vi "Lock Graph Legend in The TopRight.vi"(6 "offset":cluster{"x":i32, "y":i32}, 8 "error in (no error)":errorcluster, 11 "TabControl in":refnum<vi>) -> (0 "error out":errorcluster)   [LabVIEW 2017]
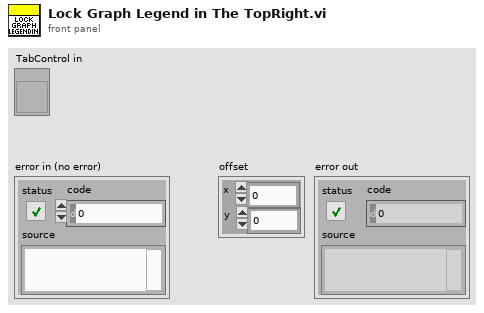
[diagram p1: front panel]
types:
  T1 = typedef "LVBoundsTypeDef.ctl" = cluster{"Width":u32, "Height":u32}
  T2 = typedef "LVPositionTypeDef.ctl" = cluster{"Left":i32, "Top":i32}
  T3 = cluster{"left":i16, "top":i16, "right":i16, "bottom":i16}
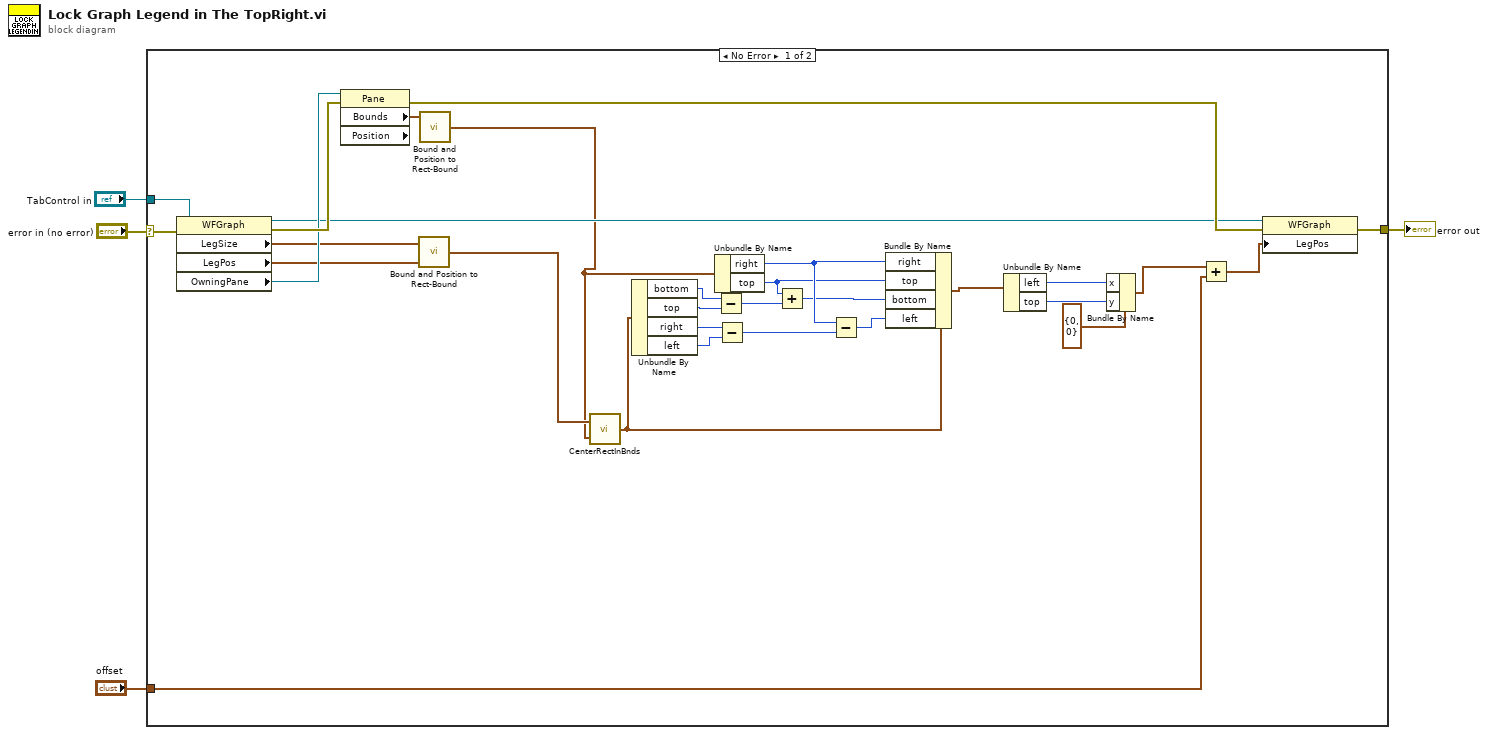
[diagram p0: block diagram]
diagram:
  n1 = case shown="No Error" "error in (no error)" {
    selector: "error in (no error)" -> [w23 w35]
    tunnel: "TabControl in" -> [w25 _]
    tunnel: [w24 w35] -> w3
    tunnel: "offset" -> [w19 _]
    frame No Error {
      n2 = property on="Property Node" class="WFGraph"(reference=w25, error in=w23) -> (reference out=w31:refnum<vi>, error out=w33:errorcluster, "LegSize"=w26:T1, "LegPos"=w27:T2, "OwningPane"=w32:refnum<vi>)
      n3 = property on="Property Node" class="Pane" props=["Bounds", "Position"](reference=w32, error in=w33) -> (error out=w34:errorcluster, "Bounds"=w28:T1)  [unwired: 2 out]
      n4 = call "Bound and Position to Rect-Bound.vi"("Position"=w27, "Bounds"=w26) -> ("Rect Bound"=w30:T3)  [unwired: 3 in]
      n5 = call "Bound and Position to Rect-Bound.vi"("Bounds"=w28) -> ("Rect Bound"=w29:T3)  [unwired: 4 in]
      n6 = call <vilib>:"CenterRectInBnds.vi"("bounds"=w29, "rect"=w30) -> ("centered rect"=w11:T3)
      n7 = Unbundle By Name(w11) -> ("bottom"=w8:i16, "top"=w9:i16, "right"=w14:i16, "left"=w15:i16)
      n8 = Unbundle By Name(w29) -> ("right"=w16:i16, "top"=w13:i16)
      n9 = Subtract(x=w8, y=w9) -> (x-y=w10:i16)
      n10 = Subtract(x=w14, y=w15) -> (x-y=w17:i16)
      n11 = Add(x=w13, y=w10) -> (x+y=w12:i16)
      n12 = Subtract(x=w16, y=w17) -> (x-y=w18:i16)
      n13 = Bundle By Name(cluster=w11, "right"=w16, "top"=w13, "bottom"=w12, "left"=w18) -> (w22:T3)
      n14 = Unbundle By Name(w22) -> ("left"=w6:i16, "top"=w7:i16)
      n15 = Bundle By Name(cluster=cluster{"x":i32, "y":i32} {"x"=0, "y"=0} ("Point"), "x"=w6, "y"=w7) -> (w21:cluster{"x":i32, "y":i32})
      n16 = Add(x=w21, y=w19) -> (x+y=w20:cluster{"x":i32, "y":i32})
      n17 = property on="Property Node" class="WFGraph"(reference=w31, error in=w34, "LegPos"=w20) -> (error out=w24:errorcluster)  [unwired: 1 out]
    }
    frame Error {
    }
  }
  "error out" <- w3
